vi "acquire.vi"(5 "Exposure Time (s)":dbl=0.004 min=0.0 step=0.001 format="%.3f", 6 "File_name":string, 7 "file path":path, 8 "error in (no error)":errorcluster, 9 "# of Frames":i32, 10 "# of spectrum per frame":i32, 11 "Camera Handle":u32) -> (0 "error out":errorcluster, 1 "?":i32[](graph), 3 "Camera Handle":u32, 4 "PyLoN Ready":bool)   [LabVIEW 2014]
uses:
  <vilib>/Utility/file.llb/Write To Spreadsheet File (I64).vi
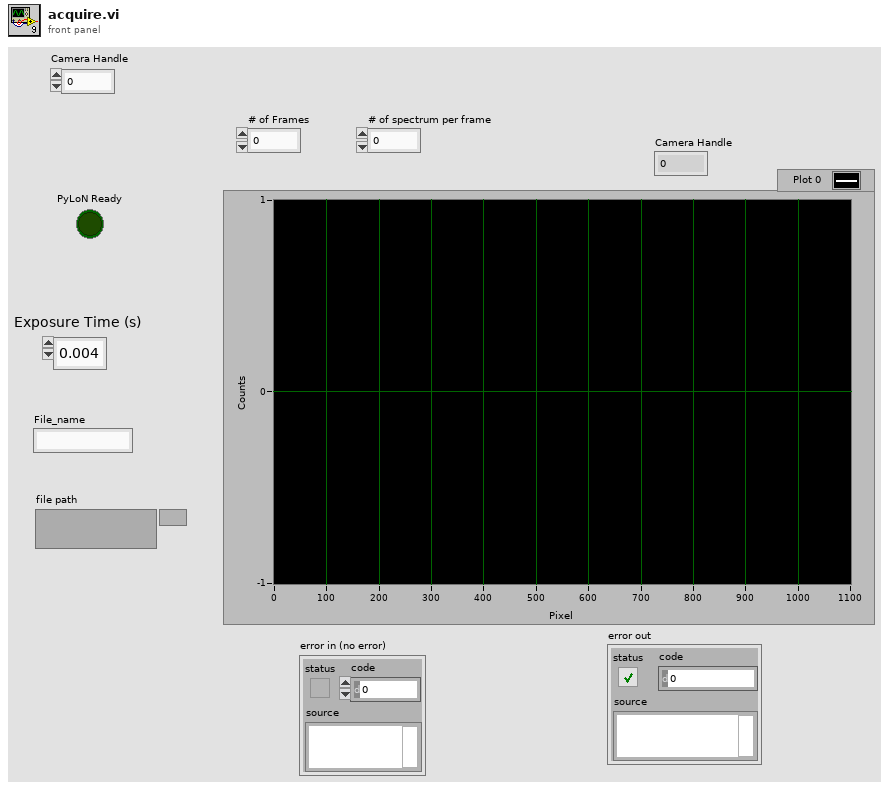
[diagram p1: front panel]
types:
  T1 = cluster{"acquire focus mode":u32, "Exposure Time (s)":dbl, i32, "Software accumulation":u32}
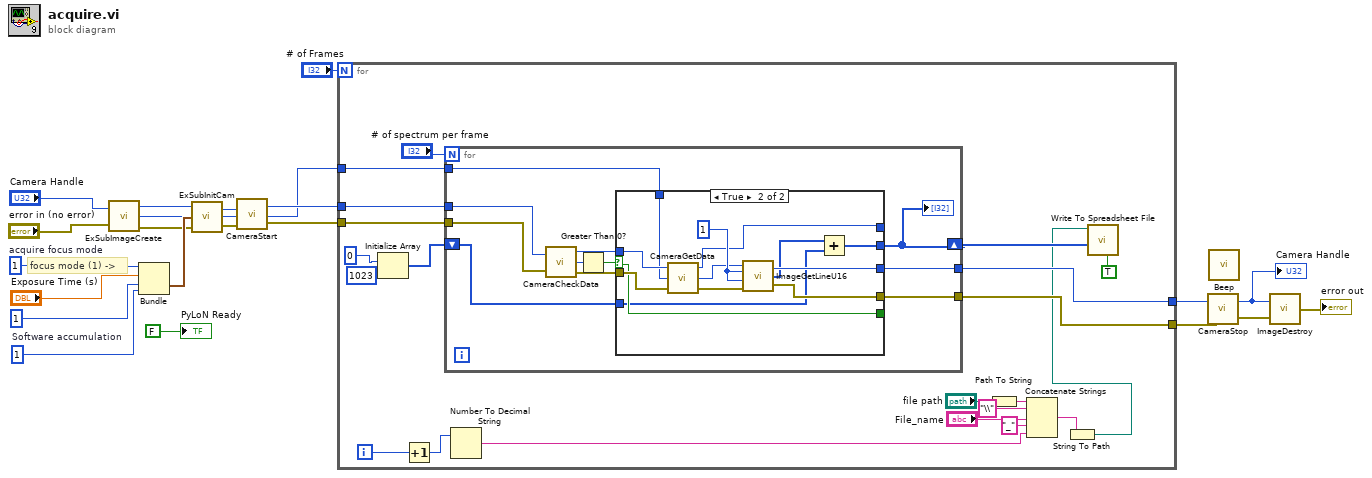
[diagram p0: block diagram]
diagram:
  w20 = u32 1  # acquire focus mode
  w19 = u32 1  # Software accumulation
  # "focus mode (1) ->"
  n1 = call "ExSubImageCreate.vi"("Camera Handle"="Camera Handle", "error in (no error)"="error in (no error)") -> ("Camera Handle"=w18:u32, "Data Handle"=w12:u32, "error out"=w17:errorcluster)
  n2 = Bundle("acquire focus mode"=w20, "Exposure Time (s)"="Exposure Time (s)", 1, "Software accumulation"=w19) -> (w21:T1)  [unwired: 1 in]
  n3 = call "ExSubInitCam.vi"("error in (no error)"=w17, "Camera Information"=w21, "Camera Handle"=w18) -> ("error out"=w16:errorcluster, "Camera Handle"=w15:u32)
  n4 = call <userlib>:"CameraStart.vi"("error in"=w16, "Camera Handle"=w15) -> ("error out"=w14:errorcluster, "Camera Handle"=w13:u32)
  n5 = for {
    N: "# of Frames" -> [_]
    tunnel: w14 -> [w42]
    tunnel: w13 -> [w41]
    tunnel: w12 -> [w40]
    tunnel: [w27] -> w5
    tunnel: [w26] -> w4
    i -> [w32]
    n6 = Initialize Array(0, 1023 ("dimension size")) -> (w23:i32[])
    n7 = Increment(x=w32) -> (x+1=w31:i32)
    n8 = for {
      N: "# of spectrum per frame" -> [_]
      tunnel: w42 -> [w53]
      tunnel: w41 -> [w52]
      tunnel: w40 -> [w51]
      shift-right: [w49] -> w38
      shift-left: w23 -> [w50]
      tunnel: [w44] -> w27
      tunnel: [w43] -> w26
      n9 = call <userlib>:"CameraCheckData.vi"("Camera Handle"=w52, "error in"=w53) -> ("Camera Handle"=w46:u32, "Number Of Frames Available"=w48:i32, "error out"=w45:errorcluster)
      n10 = Greater Than 0?(x=w48) -> (x > 0?=w47:bool)
      n11 = case shown="True" w47 {
        selector: w47 -> [w57 w69]
        tunnel: w46 -> [w55 w71]
        tunnel: w45 -> [w58 w70]
        tunnel: [w57 w69] -> _
        tunnel: [w58 w68] -> w43
        tunnel: w51 -> [w56 w62]
        tunnel: [w56 w66] -> w44
        tunnel: [w55 w65] -> _
        tunnel: [w54 w61] -> w49
        tunnel: w50 -> [w54 w59]
        frame False {
        }
        frame True {
          w67 = 1
          n12 = call <userlib>:"CameraGetData.vi"("error in"=w70, "Data Handle"=w62, "Camera Handle"=w71) -> ("error out"=w64:errorcluster, "Data Handle"=w63:u32, "Camera Handle"=w65:u32)
          n13 = call <userlib>:"ImageGetLineU16.vi"("Data Handle"=w63, "Y Position"=w67, "Z Position"=w67, "error in"=w64) -> ("Array u16"=w60:u16[], "Data Handle"=w66:u32, "error out"=w68:errorcluster)
          n14 = Add(x=w60, y=w59) -> (x+y=w61:i32[])
        }
      }
      "?" <- w49
    }
    n15 = Number To Decimal String(number=w31) -> (decimal integer string=w30:string)  [unwired: 1 in]
    n16 = Path To String(path="file path") -> (string=w36:string)
    n17 = Concatenate Strings(w36, "\\" ("string"), "File_name", "_" ("string"), w30) -> (w29:string)
    n18 = String To Path(string=w29) -> (path=w25:path)
    n19 = call-poly <vilib>:"Write To Spreadsheet File.vi"("transpose? (no:F)"=TRUE, "1D data"=w38, "file path (dialog if empty)"=w25) -> ()  [unwired: 5 in, 1 out]
  }
  n20 = call <userlib>:"CameraStop.vi"("error in"=w4, "Camera Handle"=w5) -> ("error out"=w3:errorcluster, "Camera Handle"=w1:u32)
  "Camera Handle" <- w1
  n21 = call <vilib>:"Beep.vi"() -> ()  [unwired: 12 in]
  n22 = call <userlib>:"ImageDestroy.vi"("error in"=w3, "Data handle"=w1) -> ("error out"=→"error out":errorcluster)
  "PyLoN Ready" <- FALSE ("PyLoN Ready")
